vi "Host.vi"() -> ()   [LabVIEW 2021]
uses:
  <vilib>/FPGAPlugInAG/PCIe-7857/niLvFpga_Open_PCIe-7857.vi
  <vilib>/rvi/interface/common/dynamic/niFpgaDynamicAddResources.vi
  <vilib>/rvi/interface/common/niFpgaWaitOnOcc.vi
  <vilib>/Utility/error.llb/Error Cluster From Error Code.vi
  <vilib>/rvi/errors/niLvFpgaAdjustHostInterfaceError.vi
  <vilib>/FPGAPlugInAG/Dynamic/niLvFpga_Close_Dynamic.vi
  <vilib>/rvi/interface/nirviOpenFPGA/nirviOpenFPGA.xnode
  FPGA Bitfiles/lvfpga2_FPGATarget_FPGA_J9MBVCOB9rw.lvbitx
  <vilib>/rvi/interface/nirviMethod/nirviMethod.xnode
  <vilib>/rvi/interface/nirviReadWriteControl/nirviReadWriteControl.xnode
  <vilib>/rvi/interface/nirviCloseFPGA/nirviCloseFPGA.xnode
  <vilib>/FPGAPlugInAG/Dynamic/niLvFpga_ConfigureFifo_Dynamic.vi
  <vilib>/rvi/errors/niLvFpgaMergeErrorWithErrorCode.vi
  <vilib>/FPGAPlugInAG/Dynamic/niLvFpga_ReadFifo_Dynamic.vi
  <vilib>/FPGAPlugInAG/Dynamic/niLvFpga_WriteFifo_Dynamic.vi
  NiFpgaLv.dll
  <vilib>/rvi/interface/Simulation/niFpgaSimulationCallBeginRW.vi
panel:
  out "Timed Out? 2":bool
  out "Timed Out?":bool
  in  "Stop":bool
  out "measured loop time (ms)":u32
  in  "minimum loop time (ms)":u32
  out "Data":fxp<+/-,32,16>[](array[numeric])
  out "Empty Elements Remaining":u32
  out "T2H Elements Remaining":u32
  out "maximun loop time (ms)":sgl
  in  "frame size (samples)":u32
  out "sampling interval":u32
  in  "sampling rate":sgl
  out "T2H Depth":u32
  out "H2T Depth":u32
  in  "Requested Depth":u32
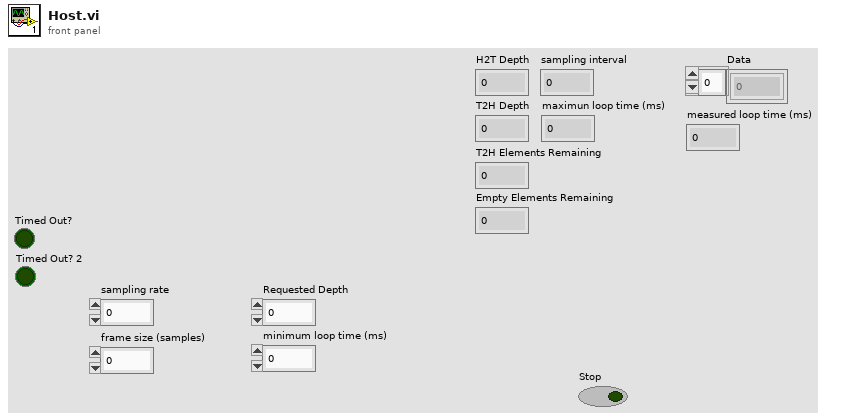
[diagram p1: front panel]
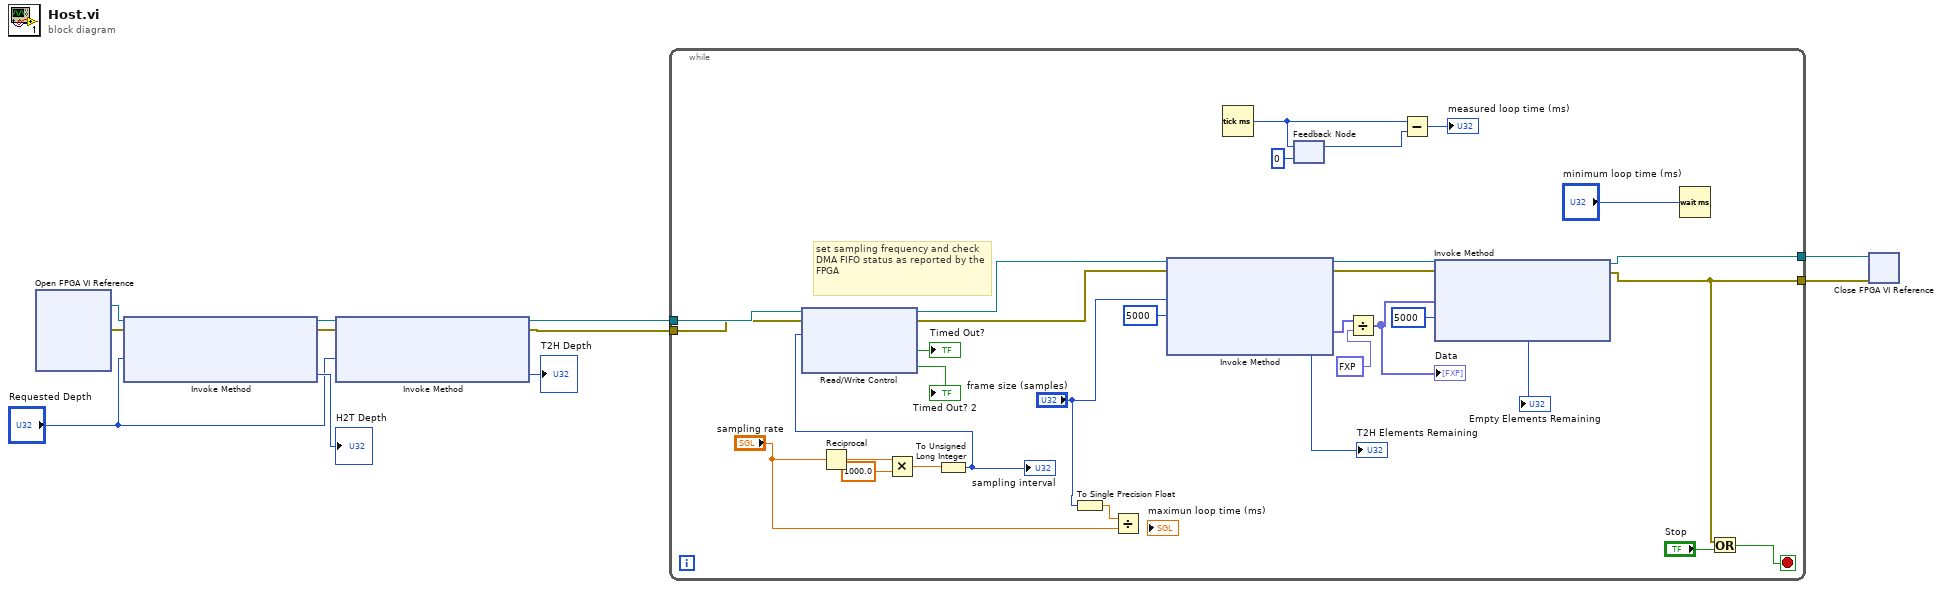
[diagram p0: block diagram]
diagram:
  n1 = xnode "Open FPGA VI Reference"() -> ("FPGA VI Reference Out"=w11:refnum<k20>, "error out"=w10:errorcluster)  [unwired: 2 in]
  n2 = xnode "Invoke Method"("FPGA VI Reference In"=w11, "error in"=w10, "Requested Depth"="Requested Depth") -> ("FPGA VI Reference Out"=w8:refnum<k20>, "error out"=w7:errorcluster, "Actual Depth"=→"H2T Depth":u32)
  n3 = xnode "Invoke Method"("FPGA VI Reference In"=w8, "error in"=w7, "Requested Depth"="Requested Depth") -> ("FPGA VI Reference Out"=w4:refnum<k20>, "error out"=w3:errorcluster, "Actual Depth"=→"T2H Depth":u32)
  n4 = while {
    tunnel: w4 -> [w42]
    tunnel: w3 -> [w41]
    tunnel: [w21] -> w2
    tunnel: [w18] -> w1
    stop <- w20 stop-if-true
    # "set sampling frequency and check DMA FIFO status as reported by the FPGA"
    n5 = Reciprocal(x="sampling rate") -> (1/x=w40:sgl)
    n6 = Multiply(x=w40, y=1000.0) -> (x*y=w38:dbl)
    n7 = To Unsigned Long Integer(number=w38) -> (unsigned 32bit integer=w37:u32)
    "sampling interval" <- w37
    n8 = xnode "Read/Write Control"("FPGA VI Reference In"=w42, "error in"=w41, "Loop Time(uSec)"=w37) -> ("FPGA VI Reference Out"=w34:refnum<k20>, "error out"=w33:errorcluster, "Timed Out?"=→"Timed Out?":bool, "Timed Out? 2"=→"Timed Out? 2":bool)
    n9 = To Single Precision Float(number="frame size (samples)") -> (single precision float=w35:sgl)
    n10 = Divide(x=w35, y="sampling rate") -> ()  [unwired: 1 out]
    n11 = xnode "Invoke Method"("FPGA VI Reference In"=w34, "error in"=w33, "Number of Elements"="frame size (samples)", "Timeout (ms)"=5000) -> ("FPGA VI Reference Out"=w30:refnum<k20>, "error out"=w29:errorcluster, "Data"=w14:fxp<+/-,32,16>[], "Elements Remaining"=→"T2H Elements Remaining":u32)
    n12 = Tick Count (ms)() -> (millisecond timer value=w24:u32)
    n13 = feedback-in #1(w24) -> ()
    n14 = feedback #1(u32 0 ("millisecond timer value")) -> (w25:u32)
    n15 = Divide(x=w14, y=fxp<+,5,7> 100.0) -> (x/y=w12:fxp<+/-,33,10>[])
    "Data" <- w12
    n16 = Subtract(x=w24, y=w25) -> (x-y=→"measured loop time (ms)":u32)
    n17 = xnode "Invoke Method"("FPGA VI Reference In"=w30, "error in"=w29, "Data"=w12, "Timeout (ms)"=5000) -> ("FPGA VI Reference Out"=w21:refnum<k20>, "error out"=w18:errorcluster, "Empty Elements Remaining"=→"Empty Elements Remaining":u32)
    n18 = Wait (ms)(milliseconds to wait="minimum loop time (ms)") -> ()  [unwired: 1 out]
    n19 = Or(x=w18, y="Stop") -> (x .or. y?=w20:bool)
  }
  n20 = xnode "Close FPGA VI Reference"("FPGA VI Reference In"=w2, "error in"=w1) -> ()  [unwired: 1 out]
